vi "sint32 decode.vi"(11 "zigzag32":u32) -> (3 "sint32":i32)   [LabVIEW 2013, in "protocol buffers encoder.lvlib"]
uses:
  protocol buffers encoder.lvlib
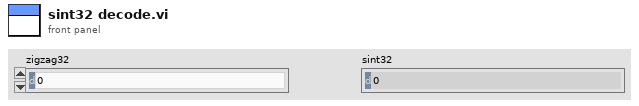
[diagram p1: front panel]
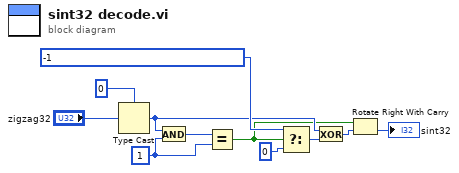
[diagram p0: block diagram]
diagram:
  w10 = 1 ("y")
  n1 = Type Cast(type=0 ("y"), x="zigzag32") -> (*(type *) &x=w5:i32)
  n2 = And(x=w5, y=w10) -> (x .and. y?=w11:i32)
  n3 = Equal?(x=w11, y=w10) -> (x = y?=w2:bool)
  n4 = Select(t=-1 ("y"), s=w2, f=0 ("t")) -> (s? t:f=w7:i32)
  n5 = Exclusive Or(1:w7, 2:w5) -> (0:w3:i32)
  n6 = Rotate Right With Carry(2:w3, 3:w2) -> (0:→"sint32":i32)  [unwired: 1 out]
